vi "StateMachineOpen.vi"(8 "error in (no error)":errorcluster, 11 "StateMachine in":refnum<class "StateMachine.lvclass">) -> (0 "error out":errorcluster, 3 "StateMachine out":refnum<class "StateMachine.lvclass">)   [LabVIEW 2018, in "StateMachine.lvclass"]
uses:
  StateMachine.lvclass
  StateMachine.lvclass/StateMachine.ctl
  <vilib>/Utility/file.llb/Read Delimited Spreadsheet (string).vi
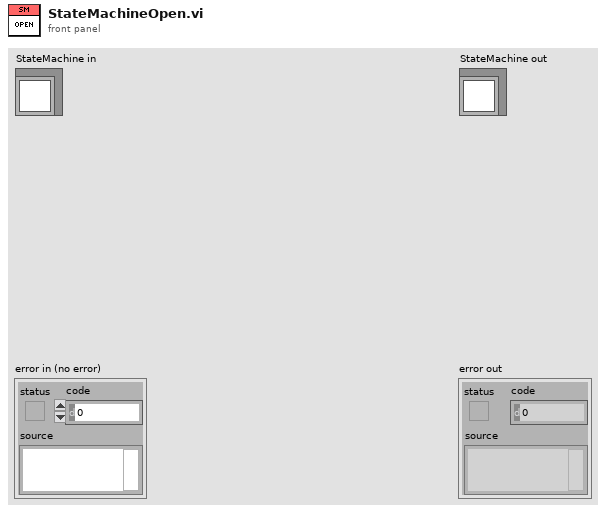
[diagram p1: front panel]
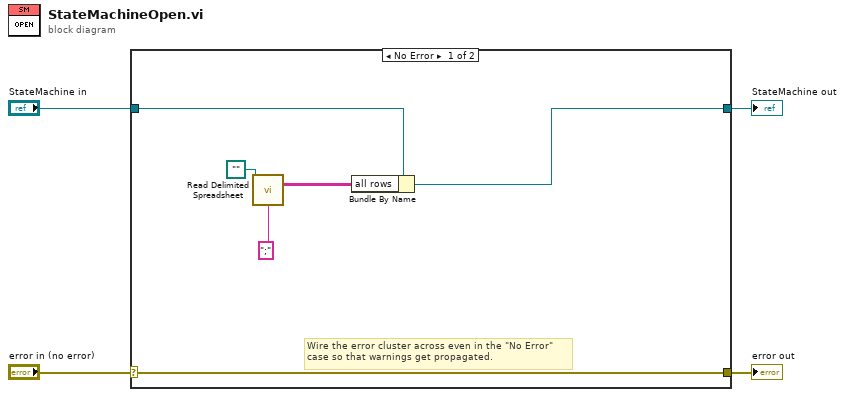
[diagram p0: block diagram]
diagram:
  n1 = case shown="No Error" "error in (no error)" {
    selector: "error in (no error)" -> [w10 w12]
    tunnel: [w10 w12] -> w3
    tunnel: [w7 w11] -> w1
    tunnel: "StateMachine in" -> [w8 w11]
    frame No Error {
      # "Wire the error cluster across even in the \"No Error\"\ncase so that warnings get propagated."
      n2 = call-poly <vilib>:"Read Delimited Spreadsheet.vi"("file path (dialog if empty)"=path "", "delimiter (\\t)"=";" ("delimiter (\\t)")) -> ("all rows"=w5:string[][])  [unwired: 8 in, 5 out]
      n3 = Bundle By Name(cluster=w8, "all rows"=w5) -> (w7:refnum<class "StateMachine.lvclass">)
    }
    frame Error {
    }
  }
  "error out" <- w3
  "StateMachine out" <- w1
